vi "Convert CAN Data (U32) to U8.vi"(0 "Data 0-3":u32 format="%032b", 7 "Data 4-7":u32 format="%032b") -> (8 "Byte Cluster":T1)   [LabVIEW 2019, in "J1939 Utilities.lvlib"]
uses:
  J1939 Utilities.lvlib
  Types/Convert CAN Data (U8) Cluster.ctl
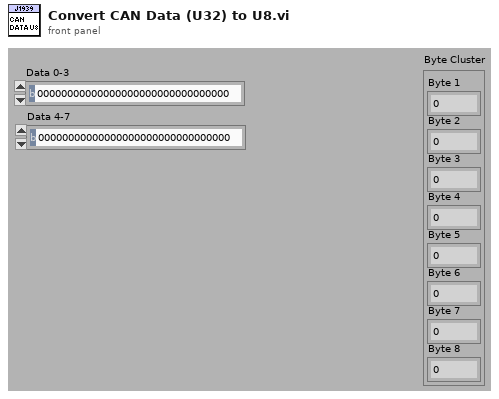
[diagram p1: front panel]
types:
  T1 = typedef "J1939 Utilities.lvlib/Convert CAN Data (U8) Cluster.ctl" = cluster{"Byte 1":u8, "Byte 2":u8, "Byte 3":u8, "Byte 4":u8, "Byte 5":u8, "Byte 6":u8, "Byte 7":u8, "Byte 8":u8}
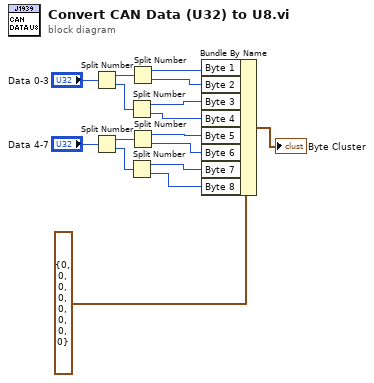
[diagram p0: block diagram]
diagram:
  n1 = Split Number(x="Data 0-3") -> (hi(x)=w16:u16, lo(x)=w13:u16)
  n2 = Split Number(x="Data 4-7") -> (hi(x)=w9:u16, lo(x)=w10:u16)
  n3 = Split Number(x=w13) -> (hi(x)=w12:u8, lo(x)=w11:u8)
  n4 = Split Number(x=w10) -> (hi(x)=w6:u8, lo(x)=w5:u8)
  n5 = Split Number(x=w16) -> (hi(x)=w15:u8, lo(x)=w14:u8)
  n6 = Split Number(x=w9) -> (hi(x)=w8:u8, lo(x)=w7:u8)
  n7 = Bundle By Name(cluster=T1 {"Byte 1"=0, "Byte 2"=0, "Byte 3"=0, "Byte 4"=0, "Byte 5"=0, "Byte 6"=0, "Byte 7"=0, "Byte 8"=0}, "Byte 1"=w15, "Byte 2"=w14, "Byte 3"=w12, "Byte 4"=w11, "Byte 5"=w8, "Byte 6"=w7, "Byte 7"=w6, "Byte 8"=w5) -> (→"Byte Cluster":T1)
